vi "example.vi"() -> ()   [LabVIEW 2021]
uses:
  <vilib>/Analysis/baseanly.llb/Mean (DBL).vi
  <vilib>/Analysis/NI_AALPro.lvlib
  <vilib>/Analysis/NI_AALBase.lvlib
panel:
  out "error out":errorcluster
  out "error out dll":errorcluster
  out "intercept dll":dbl
  out "slope dll":dbl
  out "MAE Theil-Sen dll":dbl format="%0.2f"
  out "error":i32
  out "MAE Least Square":dbl format="%0.2f"
  out "MAE Theil-Sen":dbl format="%0.2f"
  out "intercept":dbl
  out "slope":dbl
  out "XY Graph":cluster{dbl[], dbl[]}[](graph)
  out "b":dbl format="%.6g"
  out "m":dbl format="%.6g"
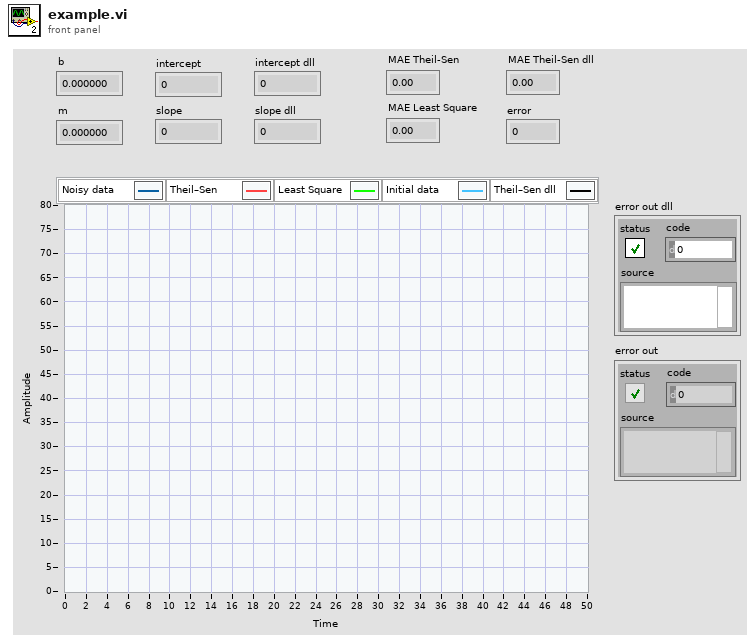
[diagram p1: front panel]
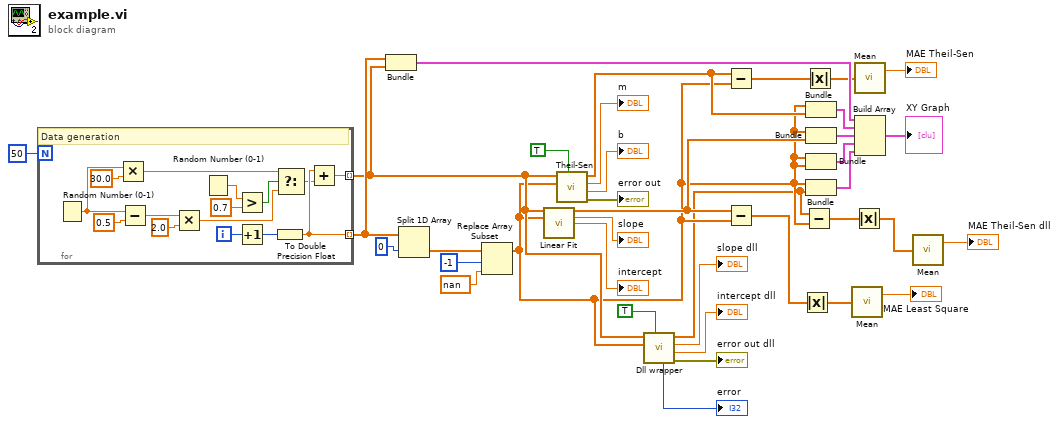
[diagram p0: block diagram]
diagram:
  n1 = for {
    N: 50 -> [_]
    tunnel: [w47] -> w14 mode=indexing
    tunnel: [w50] -> w8 mode=indexing
    i -> [w49]
    # "Data generation"
    n2 = Random Number (0-1)() -> (number: 0 to 1=w40:dbl)
    n3 = Multiply(x=w40, y=30.0 ("t")) -> (x*y=w39:dbl)
    n4 = Subtract(x=w40, y=0.5) -> (x-y=w52:dbl)
    n5 = Multiply(x=w52, y=2.0) -> (x*y=w43:dbl)
    n6 = Random Number (0-1)() -> (number: 0 to 1=w46:dbl)
    n7 = Greater?(x=w46, y=0.7) -> (0:w42:bool)
    n8 = Increment(x=w49) -> (x+1=w48:i32)
    n9 = To Double Precision Float(number=w48) -> (double precision float=w47:dbl)
    n10 = Select(t=w39, s=w42, f=w43) -> (s? t:f=w38:dbl)
    n11 = Add(x=w47, y=w38) -> (x+y=w50:dbl)
  }
  n12 = Bundle(w14, w8) -> (w36:cluster{dbl[], dbl[]})  [unwired: 1 in]
  n13 = Split 1D Array(array=w14, index=0) -> (second subarray=w12:dbl[])  [unwired: 1 out]
  n14 = Replace Array Subset(array=w12, new element=nan ("new element/subarray"), index=-1) -> (w7:dbl[])
  n15 = call <vilib>:"Linear Fit.vi"("Y"=w8, "X"=w7) -> ("Best Linear Fit"=w18:dbl[], "slope"=→"slope":dbl, "intercept"=→"intercept":dbl)  [unwired: 9 in, 2 out]
  n16 = call "Theil-Sen.vi"("match_lengths (T)"=TRUE, "input_X"=w7, "input_Y"=w8) -> ("error out"=→"error out":errorcluster, "b"=→"b":dbl, "m"=→"m":dbl, "output_Y"=w29:dbl[])  [unwired: 3 in]
  n17 = call "Dll wrapper.vi"("match_lengths (T)"=TRUE, "X"=w7, "Y"=w8) -> ("error out"=→"error out dll":errorcluster, "intercept"=→"intercept dll":dbl, "slope"=→"slope dll":dbl, "Y_out"=w6:dbl[], "error"=→"error":i32)  [unwired: 4 in]
  n18 = Subtract(x=w29, y=w7) -> (x-y=w28:dbl[])
  n19 = Subtract(x=w18, y=w7) -> (x-y=w27:dbl[])
  n20 = Absolute Value(x=w27) -> (abs(x)=w25:dbl[])
  n21 = Subtract(x=w6, y=w7) -> (x-y=w19:dbl[])
  n22 = Absolute Value(x=w28) -> (abs(x)=w26:dbl[])
  n23 = Bundle(w7, "output_Y"=w29) -> (w35:cluster{dbl[], "output_Y":dbl[]})  [unwired: 1 in]
  n24 = Bundle(w7, "Best Linear Fit"=w18) -> (w32:cluster{dbl[], "Best Linear Fit":dbl[]})  [unwired: 1 in]
  n25 = Bundle(w7, w7) -> (w33:cluster{dbl[], dbl[]})  [unwired: 1 in]
  n26 = Bundle(w7, "Y_out"=w6) -> (w22:cluster{dbl[], "Y_out":dbl[]})  [unwired: 1 in]
  n27 = call-poly <vilib>:"Mean.vi"("X"=w25) -> ("mean"=→"MAE Least Square":dbl)  [unwired: 1 out]
  n28 = Absolute Value(x=w19) -> (abs(x)=w20:dbl[])
  n29 = call-poly <vilib>:"Mean.vi"("X"=w26) -> ("mean"=→"MAE Theil-Sen":dbl)  [unwired: 1 out]
  n30 = Build Array(w36, w35, w32, w33, w22) -> (→"XY Graph":cluster{dbl[], "Y_out":dbl[]}[])
  n31 = call-poly <vilib>:"Mean.vi"("X"=w20) -> ("mean"=→"MAE Theil-Sen dll":dbl)  [unwired: 1 out]
